vi "ScriptBroadcastVI.vi"(4 "Request Name":string, 6 "EventClusterName":string, 8 "error in (no error)":errorcluster, 9 "TypeDef Path":path, 10 "Module Ref":refnum<vi>, 11 "VI in":refnum<vi>) -> (0 "error out":errorcluster)   [LabVIEW 2024, in "AddNewEvent.lvlib"]
uses:
  Event/AddNewEvent.lvlib
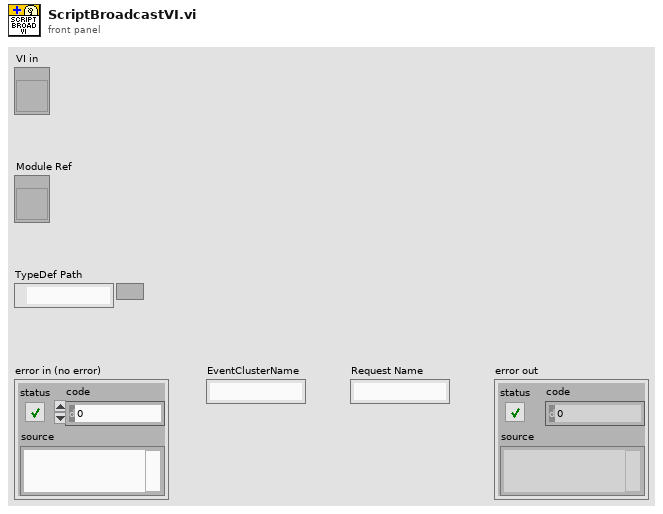
[diagram p1: front panel]
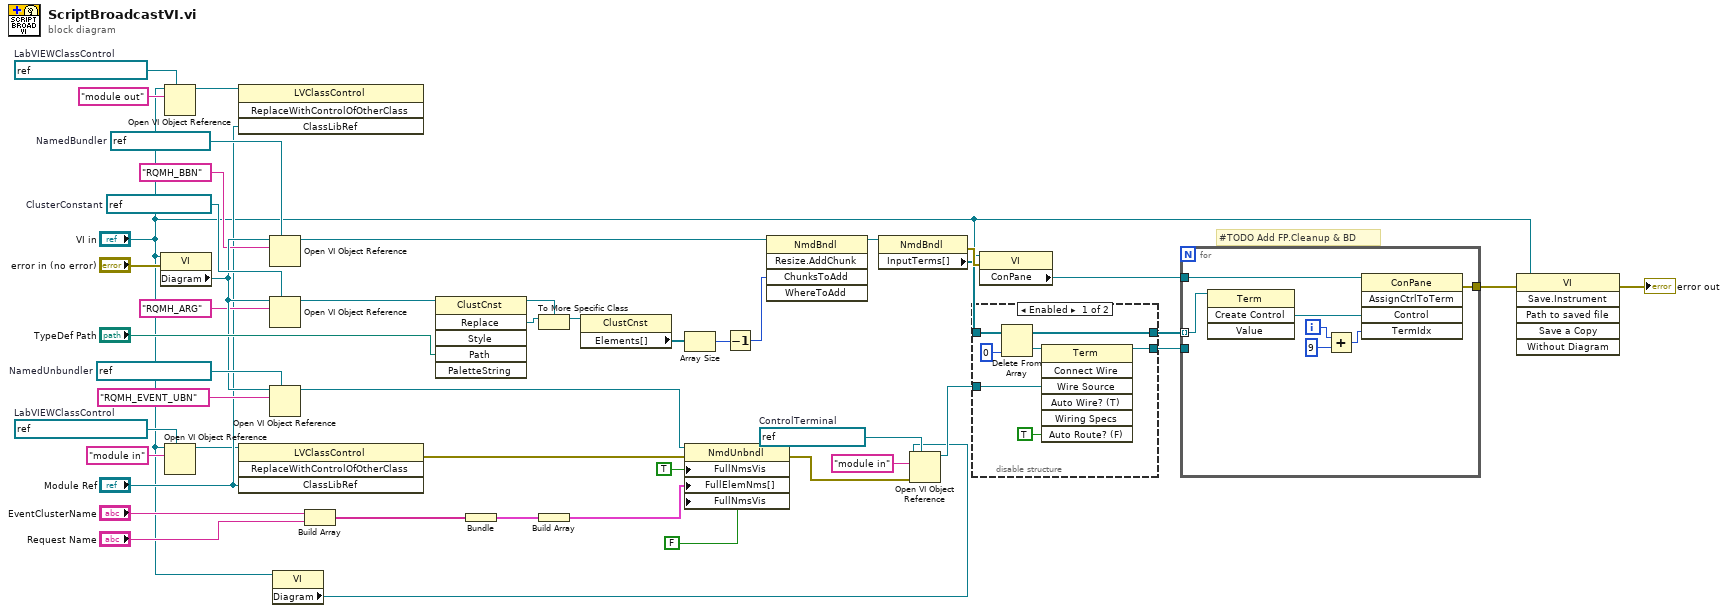
[diagram p0: block diagram]
diagram:
  w7 = refnum<vi> refnum  # ControlTerminal
  w25 = refnum<vi> refnum  # LabVIEWClassControl
  w22 = refnum<vi> refnum  # LabVIEWClassControl
  w21 = refnum<vi> refnum  # ClusterConstant
  w20 = refnum<vi> refnum  # NamedBundler
  w19 = refnum<vi> refnum  # NamedUnbundler
  # "#TODO Add FP.Cleanup & BD"
  n1 = property class="VI"(reference="VI in", error in="error in (no error)") -> ("Diagram"=w18:refnum<vi>)  [unwired: 2 out]
  n2 = Open VI Object Reference(7:w25, 10:"module out" ("name/order"), 11:"VI in") -> (3:w26:refnum<vi>)  [unwired: 1 in, 1 out]
  n3 = Open VI Object Reference(7:w22, 10:"module in" ("name/order"), 11:"VI in") -> (3:w8:refnum<vi>)  [unwired: 1 in, 1 out]
  n4 = invoke class="LVClassControl" method="ReplaceWithControlOfOtherClass"(reference=w26, "ClassLibRef"="Module Ref") -> ()  [unwired: 2 in, 4 out]
  n5 = invoke class="LVClassControl" method="ReplaceWithControlOfOtherClass"(reference=w8, "ClassLibRef"="Module Ref") -> (error out=w43:errorcluster)  [unwired: 2 in, 3 out]
  n6 = Open VI Object Reference(7:w20, 10:"RQMH_BBN" ("name/order"), 11:w18) -> (3:w33:refnum<vi>)  [unwired: 1 in, 1 out]
  n7 = Open VI Object Reference(7:w21, 10:"RQMH_ARG" ("name/order"), 11:w18) -> (3:w32:refnum<vi>)  [unwired: 1 in, 1 out]
  n8 = Open VI Object Reference(7:w19, 10:"RQMH_EVENT_UBN" ("name/order"), 11:w18) -> (3:w29:refnum<vi>)  [unwired: 1 in, 1 out]
  n9 = property class="VI"(reference="VI in") -> ("Diagram"=w3:refnum<vi>)  [unwired: 1 in, 2 out]
  n10 = Build Array("EventClusterName", "Request Name") -> (w27:string[])
  n11 = invoke class="ClustCnst" method="Replace"(reference=w32, "Path"="TypeDef Path") -> (reference out=w38:refnum<vi>, "Replace"=w36:refnum<vi>)  [unwired: 4 in, 4 out]
  n12 = Bundle(w27) -> (w28:cluster{string[]})  [unwired: 1 in]
  n13 = To More Specific Class(target class=w38, reference=w36) -> (specific class reference=w37:refnum<vi>)  [unwired: 1 in, 1 out]
  n14 = Build Array(w28) -> (w30:cluster{string[]}[])
  n15 = property class="ClustCnst"(reference=w37) -> ("Elements[]"=w34:refnum<vi>[])  [unwired: 1 in, 2 out]
  n16 = Array Size(array=w34) -> (size(s)=w35:i32)
  n17 = property class="NmdUnbndl"(reference=w29, error in=w43, "FullNmsVis"=TRUE ("Full Names Visible?"), "FullElemNms[]"=w30, "FullNmsVis"=FALSE ("Full Names Visible?")) -> (error out=w5:errorcluster)  [unwired: 1 out]
  n18 = Decrement(x=w35) -> (x-1=w39:i32)
  n19 = invoke class="NmdBndl" method="Resize.AddChunk"(reference=w33, "ChunksToAdd"=w39) -> (reference out=w40:refnum<vi>)  [unwired: 3 in, 4 out]
  n20 = property class="NmdBndl"(reference=w40) -> (error out=w46:errorcluster, "InputTerms[]"=w11:refnum<vi>[])  [unwired: 1 in, 1 out]
  n21 = Open VI Object Reference(7:w7, 8:w5, 10:"module in" ("name/order"), 11:w3) -> (3:w4:refnum<vi>)  [unwired: 1 out]
  n22 = disable-structure shown="Enabled" {
    disable-tunnel: [w52 w55] -> w12
    disable-tunnel: w11 -> [w51 w55]
    disable-tunnel: [w49 _] -> w10
    disable-tunnel: w4 -> [w48 _]
    frame Enabled {
      n23 = Delete From Array(array=w51, index=0) -> (deleted portion=w53:refnum<vi>, array with subset deleted=w52:refnum<vi>[])  [unwired: 1 in]
      n24 = invoke class="Term" method="Connect Wire"(reference=w53, "Wire Source"=w48, "Auto Route? (F)"=TRUE) -> (reference out=w49:refnum<vi>)  [unwired: 4 in, 6 out]
    }
    frame Disabled {
    }
  }
  n25 = property class="VI"(reference="VI in", error in=w46) -> ("ConPane"=w41:refnum<vi>)  [unwired: 2 out]
  n26 = for {
    tunnel: w41 -> [w62]
    tunnel: [w60] -> w42
    tunnel: w12 -> [w56] mode=indexing
    tunnel: w10 -> [_]
    i -> [w59]
    n27 = invoke class="Term" method="Create Control"(reference=w56) -> ("Create Control"=w61:refnum<vi>)  [unwired: 3 in, 3 out]
    n28 = Add(x=w59, y=9) -> (x+y=w57:i32)
    n29 = invoke class="ConPane" method="AssignCtrlToTerm"(reference=w62, "Control"=w61, "TermIdx"=w57) -> (error out=w60:errorcluster)  [unwired: 2 in, 4 out]
  }
  n30 = invoke class="VI" method="Save.Instrument"(reference="VI in", error in=w42) -> (error out=→"error out":errorcluster)  [unwired: 4 in, 5 out]
